vi "SYST_PRES.vi"(0 "VISA IN":refnum<visa-resource-name>, 5 "error in":errorcluster) -> (14 "VISA Out":refnum<visa-resource-name>, 19 "error out":errorcluster)   [LabVIEW 2018, in "PNA-X.lvlib"] (continued)
 Count (PWIN ONLY) \n1758\n\n<value> (String) Parameter Value for the specified stage 3 parameter. Use the query form \nto return the minimum and maximum values for the specified parameter. \nExamples SENS:IF:FILT:STAGe3:PAR \"C\",64 \nsense2:if:filter:stage3:parameter \"d\",0.5E-6 \nQuery Syntax SENSe<cnum>:IF:FILTer:STAGE3:PARameter? <p> \nreturns the current parameter value \nSENSe<cnum>:IF:FILTer:STAGE3:PARameter? <p>,Min \nreturns the minimum parameter value. \nSENSe<cnum>:IF:FILTer:STAGE3:PARameter? <p>,Max \nreturns the maximum parameter value. \nExamples SENS:IF:FILT:STAGe3:PAR? \"C\" \nsense2:if:filter:stage3:parameter? \"d\",min \nReturn Type Numeric \nDefault RECT: C = 1 \nPWIN: C=1E6, P=10ms, D=50us, W=50us, R=7 \nTUKEY: C=1 \nSENSe<cnum>:IF:FILTer:STAGE3:PCATalog? \n(Read-only) Returns a list of the available parameters for the currently selected filter type. \nCritical Note \nParameters \n<cnum> Existing channel number. If unspecified, <cnum> is set to 1. \nExamples SENS:IF:FILT:STAGe3:PCAT? \nsense2:if:filter:stage3:pcatalog? \nReturn Type String \nDefault Not Applicable \nSENSe<cnum>:IF:FREQuency:AUTO <bool> \n1759\n\n(Read-Write) Sets and returns the method for specifying the way the IF Frequency is determined. \nCritical Note \nParameters \n<cnum> Existing channel number. If unspecified, <cnum> is set to 1. \n<bool> (Boolean) \nON (or 1) - Automatic. PNA determines the setting for the IF frequency. \nOFF (or 0) - Manual. Use SENS:IF:FREQ to set the frequency. \nExamples SENS:IF:FREQ:AUTO 1 \nsense2:if:frequency:auto 0 \nQuery Syntax SENSe<cnum>:IF:FREQuency:AUTO? \nReturn Type Boolean \nDefault ON \nSENSe<cnum>:IF:FREQuency[:VALue] <value> \n(Read-Write) Sets and returns the IF frequency for ALL receiver paths being used for the specified \nchannel. To set this frequency, SENS:IF:FREQ:AUTO must be set to OFF (Manual). \nAlso returns the maximum and minimum allowable frequency settings. \nCritical Note \nParameters \n<cnum> Existing channel number. If unspecified, <cnum> is set to 1. \n<value> (Numeric) Frequency value. \nExamples SENS:IF:FREQ \nsense2:if:frequency \nQuery Syntax SENSe<cnum>:IF:FREQuency? \n'returns the current frequency setting \nSENSe<cnum>:IF:FREQuency? Max \n'returns the maximum allowable frequency setting \nSENSe<cnum>:IF:FREQuency? Min \n'returns the minimum allowable frequency setting \nReturn Type Numeric \nDefault 9 MHz \n1760\n\nLast Modified: \n18-Jan-2007 MX New topic \n1761\n\nSense:Mixer Commands \nPerforms Mixer setup and configuration. \nClick on a blue keyword to view the command details. \nSee Also \nExample Programs \nLearn about the Frequency Converter Application \nSynchronizing the PNA and Controller \nSCPI Command Tree \nSENSe<ch>:MIXer:APPLy \n(Write only) Applies the mixer setup settings and turns the channel ON. (Performs the same function \nas the Apply button on the mixer setup dialog box). \nParameters \n<ch> Any existing channel number. If unspecified, value is set to 1 \nExamples SENS:MIX:APPL \nQuery Syntax Not Applicable \nDefault Not Applicable \n1762\n\nSENSe<ch>:MIXer:AVOidspurs <bool> \n(Read Write) Sets and returns the state of the avoid spurs feature. Learn more about avoid spurs. \nParameters \n<ch> Any existing channel number. If unspecified, value is set to 1 \n<bool> Avoid spurs state. Choose from \n0 - Avoid spurs OFF \n1 - Avoid spurs ON \nExamples SENS:MIX:AVO \nsense2:mixer:avoidspurs 1 \nQuery Syntax SENSe<ch>:MIXer:AVOidspurs? \nReturn Type Boolean \nDefault 0 (OFF) \nSENSe<ch>:MIXer:CALCulate <char> \n(Write only) Calculates the Input, IF, or Output frequencies of the mixer setup and updates the \nchannel settings. \nParameters \n<ch> Any existing channel number. If unspecified, value is set to 1 \n<char> Mixer port to be calculated. Choose from: \n1763\n\n<char> 1st or only stage \nrequires: \nIn addition, 2nd stage \nrequires: \nINPUT \nOutput Start and Stop \nfrequencies \nLO frequency \nOutput sideband (High or \nLow) \nIF Start and Stop \nfrequencies \n2nd LO frequency \nIF sideband (High or Low) \nBoth NA \nIF Start and Stop \nfrequencies \nBoth LO frequencies \nOUTPUT \nInput Start and Stop \nfrequencies \nLO frequency \nOutput sideband (High or \nLow) \nIF Start and Stop \nfrequencies \n2nd LO frequency \nIF sideband (High or Low) \nLO_1 \nInput Start and Stop \nfrequencies \nOutput frequency \nOutput sideband (High or \nLow) \nIF Start and Stop \nfrequencies \n2nd LO frequency \nIF sideband (High or Low) \nLO_2 NA Input Start and stop \nfrequencies \n1st LO start and stop \nfrequencies \nOutput frequency \nIF sideband(High or Low \nOutput sideband(High or \nLow) \nExamples SENS:MIX:CALC Output \nQuery Syntax Not Applicable \nDefault Not Applicable \nSENSe<ch>:MIXer:LOAD <name> \n1764\n\n(Write-only) Loads a previously-configured mixer attributes file (.mxr) \nParameters \n<ch> Any existing channel number. If unspecified, value is set to 1. \n<name> Path and file name (including .mxr extension) to load. \nExamples SENSe:MIXer:LOAD \"C:\\Program Files\\Agilent\\Network \nAnalyzer\\Documents\\Mixer\\MyMixer.mxr\" \nDefault Not Applicable \nSENSe<ch>:MIXer:SAVE <name> \n(Write-only) Saves the settings for the mixer/converter test setup to a mixer attributes file. \nParameters \n<ch> Any existing channel number. If unspecified, value is set to 1. \n<name> Path and file name (including .mxr extension) to save. \nExamples SENSe:MIXer:SAVE \"C:\\Program Files\\Agilent\\Network \nAnalyzer\\Documents\\Mixer\\MyMixer.mxr\" \nDefault Not Applicable \nSENSe<ch>:MIXer:STAGe <n> \n(Read-Write) Number of IF stages of the mixer. \nParameters \n<ch> Any existing channel number. If unspecified, value is set to 1. \n<n> Number of stages. Choose either 1 or 2 \nExamples SENSe:MIX:STAG 2 \nSENSe:MIXer:STAGE 1 \nQuery Syntax SENSe<ch>:MIXer:STAGe? \nReturn Type Numeric \nDefault 1 \nSENSe<ch>:MIXer:IF:FREQuency:DENominator <num> \n1765\n\n(Read-Write) Sets or returns the denominator value of the IF Fractional Multiplier. \nParameters \n<ch> Any existing channel number. If unspecified, value is set to 1. \n<num> Denominator value. \nExamples SENSe:MIX:IF:FREQ:DEN 5 \nSENSe2:MIXer:IF:FREQ:DENominator 4 \nQuery Syntax SENSe<ch>:MIXer:IF:FREQuency:DENominator? \nReturn Type Numeric \nDefault Not Applicable \nSENSe<ch>:MIXer:IF:FREQuency:FIXed <num> \n(Read-Write) Sets or returns the fixed frequency of the IF.. \nParameters \n<ch> Any existing channel number. If unspecified, value is set to 1. \n<num> Frequency. \nExamples SENSe:MIXer:IF:FREQ:FIXed 1e9 \nSENSe2:MIXer:IF:FREQ:FIXed 1000000000 \nQuery Syntax SENSe<ch>:MIXer:IF:FREQuency:FIXed? \nReturn Type Numeric \nDefault Not Applicable \nSENSe<ch>:MIXer:IF:FREQuency:NUMerator <num> \n(Read-Write) Sets or returns the numerator value of the IF Fractional Multiplier. \nParameters \n<ch> Any existing channel number. If unspecified, value is set to 1. \n<num> Numerator value of the IF fractional multiplier \nExamples SENSe:MIX:IF:FREQ:NUM 4 \nSENSe2:MIXer:IF2:FREQ:NUMerator 3 \nQuery Syntax SENSe<ch>:MIXer:IF:FREQuency:NUMerator? \nReturn Type Numeric \nDefault Not Applicable \n1766\n\nSENSe<ch>:MIXer:IF:FREQuency:SIDeband <char> \n(Read-Write) Sets or returns the value of the IF sideband. \nParameters \n<ch> Any existing channel number. If unspecified, value is set to 1. \n<char> Sideband value. Choose from \nLOW - Low or Difference (-) \nHIGH - High or Sum (+) \nExamples SENS:MIX:IF:FREQ:SIDE LOW \nSENSe2:MIXer:IF:FREQ:SIDEband HIGH \nQuery Syntax SENSe<ch>:MIXer:IF:FREQuency:SIDeband? \nReturn Type Character \nDefault LOW \nSENSe<ch>:MIXer:IF:FREQuency:STARt <num> \n(Read-Write) Sets or returns the IF start frequency value of the mixer. \nParameters \n<ch> Any existing channel number. If unspecified, value is set to 1. \n<num> IF Start Frequency value \nExamples SENS:MIX:IF:FREQ:STAR 1e9 \nSENSe2:MIXer:IF:FREQ:STARt 1000000000 \nQuery Syntax SENSe<ch>:MIXer:IF:FREQuency:STARt? \nReturn Type Numeric \nDefault Not Applicable \nSENSe<ch>:MIXer:IF:FREQuency:STOP <num>\n1767\n\n(Read-Write) Sets or returns the stop frequency value of the mixer IF frequency. \nParameters \n<ch> Any existing channel number. If unspecified, value is set to 1. \n<num> IF Stop Frequency value \nExamples SENS:MIX:IF:FREQ:STOP 2e9 \nSENSe2:MIXer:IF:FREQ:STOP 2000000000 \nQuery Syntax SENSe<ch>:MIXer:IF:FREQuency:STOP? \nReturn Type Numeric \nDefault Not Applicable \nSENSe<ch>:MIXer:INPut:FREQuency:DENominator <value> \n(Read-Write) Sets or returns the denominator value of the Input Fractional Multiplier. \nParameters \n<ch> Any existing channel number. If unspecified, value is set to 1. \n<value> Input denominator value. \nExamples SENS:MIX:INP:FREQ:DEN 5 \nSENS2:MIXer:INPut:FREQ:DENominator 4 \nQuery Syntax SENSe<ch>:MIXer:INPut:FREQuency:DENominator? \nReturn Type Numeric \nDefault Not Applicable \nSENSe<ch>:MIXer:INPut:FREQuency:FIXed<value> \n(Read-Write) Sets or returns the fixed frequency of the input. \nParameters \n<ch> Any existing channel number. If unspecified, value is set to 1. \n<value> Input frequency. \nExamples SENSe:MIXer:INPut:FREQ:FIXed 1e9 \nSENSe2:MIXer:INPut:FREQ:FIXed 1000000000 \nQuery Syntax SENSe<ch>:MIXer:INPut:FREQuency:FIXed? \nReturn Type Numeric \nDefault Not Applicable \n1768\n\nSENSe<ch>:MIXer:INPut:FREQuency:MODE <char> \n(Read-Write) Sets or returns the Input sweep mode. \nParameters \n<ch> Any existing channel number. If unspecified, value is set to 1. \n<char> Input sweep mode. Choose either FIXED or SWEPT \nExamples SENS:MIX:INP:FREQ:MODE FIXED \nSENSe2:MIXer:INP:FREQ:MODE swept \nQuery Syntax SENSe<ch>:MIXer:INPut:FREQuency:MODE? \nReturn Type Character \nDefault Fixed \nSENSe<ch>:MIXer:INPut:FREQuency:NUMerator <value> \n(Read-Write) Sets or returns the numerator value of the Input Fractional Multiplier. \nParameters \n<ch> Any existing channel number. If unspecified, value is set to 1. \n<value> Input numerator value. \nExamples SENS:MIX:INP:FREQ:NUM 3 \nSENSe2:MIXer:INPut:FREQ:NUMerator 1 \nQuery Syntax SENSe<ch>:MIXer:INPut:FREQ:NUMerator? \nReturn Type Numeric \nDefault Not Applicable \nSENSe<ch>:MIXer:INPut:FREQuency:STARt <value> \n1769\n\n(Read-Write) Sets or returns the Input start frequency value of the mixer. \nParameters \n<ch> Any existing channel number. If unspecified, value is set to 1. \n<value> Input Start frequency \nExamples SENS:MIX:INP:FREQ:STAR 1e9 \nSENSe2:MIXer:INPut:FREQ:STARt 1000000000 \nQuery Syntax SENSe<ch>:MIXer:INPut:FREQuency:STARt? \nReturn Type Numeric \nDefault Not Applicable \nSENSe<ch>:MIXer:INPut:FREQuency:STOP <value> \n(Read-Write) Sets or returns the Input stop frequency value of the mixer. \nParameters \n<ch> Any existing channel number. If unspecified, value is set to 1. \n<value> Input stop frequency \nExamples SENS:MIX:INP:FREQ:STOP 2e9 \nSENSe2:MIXer:INPut:FREQ:STOP 2000000000 \nQuery Syntax SENSe<ch>:MIXer:INPut:FREQuency:STOP? \nReturn Type Numeric \nDefault Not Applicable \nSENSe<ch>:MIXer:INPut:POWer <value> \n(Read-Write) Sets or returns the value of the Input Power. \nParameters \n<ch> Any existing channel number. If unspecified, value is set to 1. \n<value> Input power in dBm. \nExamples SENS:MIX:INP:POW 9 \nSENSe2:MIXer:INPut:POWer 5 \nQuery Syntax SENSe<ch>:MIXer:INPut:POWer? \nReturn Type Numeric \nDefault Not Applicable \n1770\n\nSENSe<ch>:MIXer:INPut:POWer:USENominal <bool> \n(Read-Write) Toggles the Nominal Incident Power setting ON and OFF. This setting is ONLY to be \nused with SMC measurements, not VMC. Learn more about Nominal Incident Power. \nParameters \n<ch> Any existing channel number. If unspecified, value is set to 1. \n<value> (boolean) - Nominal Incident Power State. Choose from: \nTrue (1) - Turn nominal incident power ON \nFalse (0) - Turn nominal incident power OFF \nExamples SENS:MIX:INP:POW:USEN 1 \nSENSe2:MIXer:INPut:POWer:USENominal false \nQuery Syntax SENSe<ch>:MIXer:INPut:POWer:USENominal? \nReturn Type Boolean \nDefault False \nSENSe<ch>:MIXer:LO<n>:FREQuency:DENominator <value> \n(Read-Write) Sets or returns the denominator value of the LO Fractional Multiplier. \nParameters \n<ch> Any existing channel number. If unspecified, value is set to 1. \n<n> LO stage number. Choose 1 or 2. \n<value> LO denominator. \nExamples SENS:MIX:LO:FREQ:DEN 5 \nSENSe2:MIXer:LO2:FREQ:DENominator 4 \nQuery Syntax SENSe<ch>:MIXer:LO<n>:FREQuency:DENominator? \nReturn Type Numeric \nDefault 1 \nSENSe<ch>:MIXer:LO<n>:FREQuency:FIXed <value> \n1771\n\n(Read-Write) Sets or returns the fixed frequency of the specified mixer LO. \nParameters \n<ch> Any existing channel number. If unspecified, value is set to 1. \n<n> LO stage number. Choose 1 or 2 \n<value> LO frequency. \nExamples SENS:MIX:LO:FREQ:FIX 1e9 \nSENSe2:MIXer:LO2:FREQ:FIXed 1000000000 \nQuery Syntax SENSe<ch>:MIXer:LO<n>:FREQuency:FIXed? \nReturn Type Numeric \nDefault Not Applicable \nSENSe<ch>:MIXer:LO<n>:FREQuency:ILTI <bool> \n(Read-Write) Specifies whether to use the Input frequency that is greater than the LO or less than \nthe LO. To learn more, see the mixer setup dialog box help. \nParameters \n<ch> Any existing channel number. If unspecified, value is set to 1. \n<n> LO stage number. Choose 1 or 2 \n<bool> True (1) - Use the Input that is Greater than the specified LO. \nFalse (0) - Use the Input that is Less than the specified LO. \nExamples SENS:MIX:LO1:FREQ:ILTI 1 \nsense2:mixer:lo2:frequency:ilti true \nQuery Syntax SENSe<ch>:MIXer:LO<n>:FREQuency:ILTI? \nReturn Type Boolean \nDefault False \nSENSe<ch>:MIXer:LO<n>:FREQuency:MODE <char> \n1772\n\n(Read-Write) Sets or returns the LO sweep mode. \nParameters \n<ch> Any existing channel number. If unspecified, value is set to 1. \n<n> LO stage number. Choose 1 or 2 \n<char> LO sweep mode. Choose either FIXED or SWEPT \nExamples SENS:MIX:LO:FREQ:MODE FIXED \nSENSe2:MIXer:LO2:FREQ:MODE swept \nQuery Syntax SENSe<ch>:MIXer:LO<n>:FREQuency:MODE? \nReturn Type Character \nDefault Fixed \nSENSe<ch>:MIXer:LO<n>:FREQuency:NUMerator <value> \n(Read-Write) Sets or returns the numerator value of the LO Fractional Multiplier. \nParameters \n<ch> Any existing channel number. If unspecified, value is set to 1. \n<n> LO stage number. Choose 1 or 2 \n<value> LO Numerator. \nExamples SENS:MIX:LO:FREQ:NUM 5 \nSENSe2:MIXer:LO2:FREQ:NUMerator 4 \nQuery Syntax SENSe<ch>:MIXer:LO<n>:FREQuency:NUMerator? \nReturn Type Numeric \nDefault Not Applicable \nSENSe<ch>:MIXer:LO<n>:FREQuency:STARt <value> \n1773\n\n(Read-Write) Sets or returns the LO start frequency value. \nParameters \n<ch> Any existing channel number. If unspecified, value is set to 1. \n<n> LO stage number. Choose 1 or 2 \n<value> LO Start Frequency in Hertz. \nExamples SENS:MIX:LO:FREQ:STAR 5E9 \nQuery Syntax SENSe<ch>:MIXer:LO<n>:FREQuency:STARt? \nReturn Type Numeric \nDefault Not Applicable \nSENSe<ch>:MIXer:LO<n>:FREQuency:STOP <value> \n(Read-Write) Sets or returns the LO stop frequency value. \nParameters \n<ch> Any existing channel number. If unspecified, value is set to 1. \n<n> LO stage number. Choose 1 or 2 \n<value> LO Stop Frequency in Hertz. \nExamples SENS:MIX:LO:FREQ:STOP 5E9 \nQuery Syntax SENSe<ch>:MIXer:LO<n>:FREQuency:STOP? \nReturn Type Numeric \nDefault Not Applicable \nSENSe<ch>:MIXer:LO<n>:NAME <value> \n1774\n\n(Read-Write) Sets or returns the name of the previously-configured external LO source. The external \nLO source must be configured and calibrated manually; there are no programming commands to \naccomplish this. The source must also be properly connected. \nParameters \n<ch> Any existing channel number. If unspecified, value is set to 1. \n<n> LO stage number. Choose 1 or 2. \n<value> External LO source name \nExamples SENS:MIX:LO:NAME \"MySource\" \nQuery Syntax SENSe<ch>:MIXer:LO<n>:NAME? \nReturn Type String \nDefault Not Controlled \nSENSe<ch>:MIXer:LO<n>:POWer <value> \n(Read-Write) Sets or returns the value of the LO Power. \nParameters \n<ch> Any existing channel number. If unspecified, value is set to 1. \n<n> LO stage. Choose 1 or 2 \n<value> LO Power in dBm \nExamples SENS:MIX:LO:POW 9 \nQuery Syntax SENSe<ch>:MIXer:LO<n>:POWer? \nReturn Type Numeric \nDefault Not Applicable \nSENSe<ch>:MIXer:OUTPut:FREQuency:FIXed <value> \n1775\n\n(Read-Write) Sets or returns the output fixed frequency of the mixer. \nParameters \n<ch> Any existing channel number. If unspecified, value is set to 1. \n<value> Output fixed frequency in Hertz. \nExamples SENS:MIX:OUTP:FREQ:FIX 5e9 \nQuery Syntax SENSe<ch>:MIXer:OUTPut:FREQuency:FIXed? \nReturn Type Numeric \nDefault Not Applicable \nSENSe<ch>:MIXer:OUTPut:FREQuency:MODE <char> \n(Read-Write) Sets or returns the Output sweep mode. \nParameters \n<ch> Any existing channel number. If unspecified, value is set to 1. \n<char> Output sweep mode. Choose either FIXED or SWEPT \nExamples SENS:MIX:OUT:FREQ:MODE FIXED \nSENSe2:MIXer:OUTput:FREQuency:MODE swept \nQuery Syntax SENSe<ch>:MIXer:OUTPut:FREQuency:MODE? \nReturn Type Character \nDefault Fixed \nSENSe<ch>:MIXer:OUTPut:FREQuency:SIDeband <value> \n1776\n\n(Read-Write) Sets or returns the value of the output sideband. \nParameters \n<ch> Any existing channel number. If unspecified, value is set to 1. \n<value> Boolean Sideband value. Choose from \nLOW - Low or Difference (-) \nHIGH - High or Sum (+) \nExamples SENS:MIX:OUTP:FREQ:SIDe LOW \nSENSe2:MIXer:OUTPut:FREQ:SIDeband HIGH \nQuery Syntax SENSe<ch>:MIXer:OUTPut:FREQuency:SIDeband? \nReturn Type Character \nDefault LOW \nSENSe<ch>:MIXer:OUTPut:FREQuency:STARt <value> \n(Read-Write) Sets or returns the Output start frequency of the mixer. \nParameters \n<ch> Any existing channel number. If unspecified, value is set to 1. \n<value> Output start frequency \nExamples SENS:MIX:OUTP:FREQ:STAR 1e9 \nSENSe2:MIXer:OUTPut:FREQ:STARt 1000000000 \nQuery Syntax SENSe<ch>:MIXer:OUTPut:FREQuency:STARt? \nReturn Type Numeric \nDefault Not Applicable \nSENSe<ch>:MIXer:OUTPut:FREQuency:STOP <value> \n1777\n\n(Read-Write) Sets or returns the Output stop frequency of the mixer. \nParameters \n<ch> Any existing channel number. If unspecified, value is set to 1. \n<value> Output stop frequency \nExamples SENS:MIX:OUTP:FREQ:STOP 1e9 \nSENSe2:MIXer:OUTPut:FREQ:STOP 1000000000 \nQuery Syntax SENSe<ch>:MIXer:OUTPut:FREQuency:STOP? \nReturn Type Numeric \nDefault Not Applicable \n1778\n\nSense:Multiplexer Commands \nControls External Test Sets (N44xx, E5091A, and Special Opts). \nClick on a blue keyword to view the command details. \nRed commands are superseded. \nSee Also \nSee an example program using these commands. \nLearn about External Test Set Control \nSynchronizing the PNA and Controller \nSCPI Command Tree \nSENSe:MULTiplexer<id>:ADDRess <address> \n(Read-Write) Sets and returns the address for the external test set at the specified ID. This command \nshould be immediately preceded by the SENSe:MULT:TYPE command. \nParameters \n<id> Id of the external test set. If unspecified, Id is assumed to be 1. Must be \npreviously set by the SENSe:MULT:TYPE command. \n<address> Integer The test set address. \nFor a GPIB test set (N44xx and some specials), this is the GPIB address. \nFor a test set I/O test set (some specials), it is the position of the test set in the chain \n(starting at 0). \nFor USB test sets (E5091A), the address is set by DIP switches on the rear panel. \n1779\n\nExamples SENS:MULT1:TYPE \"Z5623A_K66\" ' use K66 test set, and reference it \nthrough ID 1 \nSENS:MULT1:ADDR 0 ' first test set in sequence \n' All subsequent commands using SENS:MULT1 will refer to this \ntest set \nQuery Syntax SENSe:MULTiplexer<id>:ADDRess? \nReturn Type Numeric \nDefault Not Applicable \nSENSe<cnum>:MULTiplexer<id>:ALLPorts <string> \n(Read-Write) Sets or gets the port selections for all available ports on the specified channel. \nParameters \n<cnum> Any existing channel number. If unspecified, value is set to 1. \n<id> Id of the external test set. If unspecified, Id is assumed to be 1. Must be \npreviously set by the SENSe:MULT:TYPE command. \n<string> Comma-separated list of port selections, one for each port. Each port selection \nmust correspond to one of the values returned by SENS:MULT:PORT:CAT?. \nDo NOT include + and - . \nExamples ' for channel 5 and test set 1, set port 1 to T1, \n' port 2 to A, port 3 to R2+, port 4 to R3-. \nSENS5:MULT1:ALLP \"T1,A,R2,R3 \" \nQuery Syntax SENSe<cnum>:MULTiplexer<id>:ALLPorts? \nReturn Type STRING \nDefault Not Applicable \nSENSe:MULTiplexer:CATalog? \n(Read-Only) Returns a comma-separated list of the external test sets models that are currently \nsupported. Choose one of these items to send SENS:MULT1:TYPE. \nExamples SENS:MULT:CAT? \nReturn Type String \nDefault Not Applicable \n1780\n\nSENSe:MULTiplexer<id>:COUNt? \n(Read-Only) Returns the total number of ports of the specified test set. \nReturns 0 if no test set is connected (GPIB test sets only). \nParameters \n<id> Id of the external test set. If unspecified, Id is assumed to be 1. Must be \npreviously set by the SENSe:MULT:TYPE command. \nExamples SENS:MULT1:COUN? \nsense:multiplexer2:count? \nReturn Type Numeric \nDefault Not Applicable \nSENSe:MULTiplexer<id>:DISPlay[:STATe] <bool> \n(Read-Write) Turns ON and OFF the display of the test set control status bar. This status bar indicates \nthe test set that is being controlled and the current port mappings. This setting is turned ON \nautomatically when the test set is enabled. \nParameters \n<id> Id of the external test set. If unspecified, Id is assumed to be 1. Must be \npreviously set by the SENSe:MULT:TYPE command. \n<bool> ON(1) Turns ON the display. \nOFF (0) Turns OFF the display. \nExamples SENS:MULT1:DISP 1 \nsense:multiplexer2:display:state on \nQuery Syntax SENSe:MULTiplexer<id>:DISPlay[:STATe]? \nReturn Type Boolean \nDefault OFF (0) \nSENSe:MULTiplexer<id>:INCount? \n1781\n\n(Read-Only) Returns the number of input ports for the specified test set. \nFor test sets such as the E5091A that do NOT use jumper cables to route the stimulus and response signals, \nthis command returns the number of test set ports that can be connected to the PNA. \nFor test sets that DO use jumper cables to route the stimulus and response signals, such as the N44xx, the \nreturn value is not valid. \nParameters \n<id> Id of the external test set. If unspecified, Id is assumed to be 1. Must be \npreviously set by the SENSe:MULT:TYPE command. \nExamples SENS3:MULT1:INC? ' returns the number of input ports for test \nset 1 on channel 3 \nReturn Type Numeric \nDefault Not Applicable \nSENSe<cnum>:MULTiplexer:LABel <string> \n(Read-Write) Sets and returns the display label for the testset on the specified channel. The label \nappears in a status bar at the bottom of the PNA display when SENS:MULT:DISP is set to TRUE. \nParameters \n<cnum> Any existing channel number. If unspecified, value is set to 1. \n<string> Display label text. \nExamples SENS3:MULT:LAB 'High-power output' \nQuery Syntax SENSe<cnum>:MULTiplexer:LABel? \nReturn Type String \nDefault Not Applicable \nSENSe<cnum>:MULTiplexer<id>:OUTPut[:DATa] <num> \n1782\n\n(Read-Write) Sets or returns the control line value for the specified channel. \nParameters \n<cnum> Any existing channel number. If unspecified, value is set to 1. \n<id> Id of the external test set. If unspecified, Id is assumed to be 1. Must be \npreviously set by the SENSe:MULT:TYPE command. \n<numr> An integer specifying the decimal value of the control line. Values are obtained \nby adding weights from the following table that correspond to individual lines. \nHIGH =1; LOW=0. \nLine Weight \n1 1 \n2 2 \n3 4 \n4 8 \n5 16 \n6 32 \n7 64 \n8 128 \n0 - Sets all lines low \n255 - Sets all lines high \nExamples SENS3:MULT1:OUTP 48 'For test set 1 on channel 3, sets lines 5 \nand 6 to HIGH state; all other lines are set to LOW state. \nQuery Syntax SENSe<cnum>:MULTiplexer<id>:OUTPut[:DATa]? \nReturn Type Numeric \nDefault Not Applicable \nSENSe:MULTiplexer<id>:PORT<pnum>CATalog? \n1783\n\n(Read-Only) Returns a comma-separated list of valid port selections for the specified port. \nParameters \n<id> Id of the external test set. If unspecified, Id is assumed to be 1. Must be \npreviously set by the SENSe:MULT:TYPE command. \n<pnum> Integer - Input port number for which to return valid Output port selections. \nRead the number of input ports for the test set using SENS:MULT:INCount? \nExamples SENS:MULT1:PORT3:CAT? ' returns the valid port selections for \nport 3 \nReturn Type String \nDefault Not Applicable \nSENSe<cnum>:MULTiplexer<id>:PORT<logi>SELect <phys> \n(Write-Only) Sets and returns a port mapping for a single port. If this command creates a conflict with \nan existing port, the PNA will resolve the conflict. \nNote: This command is currently not supported for the Z5623AK44. \nParameters \n<cnum> Channel number of the measurement. If unspecified, value is set to 1. \n<id> Id of the external test set. If unspecified, Id is assumed to be 1. Must be \npreviously set by the SENSe:MULT:TYPE command. \n<logi> Integer - Logical port number. \n<string> String - Physical port number. \nExamples SENS:MULT1:PORT3:SEL \"4\" 'sets logical port 3 to physical port \n4. \nReturn Type String \nDefault Not Applicable \nSENSe:MULTiplexer<id>:STATe <bool> \n1784\n\n(Read-Write) Enables and disables (ON/OFF) the port mapping and control line output of the \nspecified test set. \nIf the specified test set is not connected or not ON, then setting State ON will report an error. All other \nproperties can be set when the test set is not connected. \nWhen this command is set to ON, then the display of the test set status bar (SENS:MULT:DISP) is \nalso set to ON. \nParameters \n<id> Id of the external test set. If unspecified, Id is assumed to be 1. Must be \npreviously set by the SENSe:MULT:TYPE command. \n<bool> ON(1) Enables test set control. \nOFF (0) Disables test set control. \nExamples SENS:MULT1:STAT 1 \nsense2:multiplexer2:state on \nQuery Syntax SENSe<cnum>:MULTiplexer<id>:STATe? \nReturn Type Boolean \nDefault OFF (0) \nSENSe<cnum>:MULTiplexer<id>:TSET9:OUTPut[:DATA] <data> Superseded \nNote: This command is replaced with SENS:MULT:OUTP \n(Read-Write) Sets the control lines of the specified E5091A. Control lines, provided through a \nE5091A front panel connector, are used to control external equipment such as a part handler. See your \nE5091A documentation to learn more about control lines. \nParameters \n<cnum> Channel number of the measurement. If unspecified, value is set to 1. \n<id> Id of the E5091A test set. Choose from 1 or 2. Learn how to set ID value. \n<data> Data value used to set control lines. Values are obtained by adding weights \nfrom the following table that correspond to individual lines. HIGH =1; \nLOW=0. \n1785\n\nLine Weight \n1 1 \n2 2 \n3 4 \n4 8 \n5 16 \n6 32 \n7 64 \n8 128 \n0 - Sets all lines low \n255 - Sets all lines high \nExamples 'The following sets line 3 and 4 high. All other lines low. \nSENS:MULT1:TSET9:OUTP 12 \nQuery Syntax SENSe<cnum>:MULTiplexer<id>:TSET9:OUTPut[:DATA]? \nReturn Type Numeric \nDefault 0 \nSENSe<cnum>:MULTiplexer<id>:TSET9:PORT1 <char> Superseded \nNote: This command is replaced with SENS:MULT:ALLPorts which sets ALL ports to the specified \noutputs. \n(Read-Write) Switches Port 1 of the specified E5091A to one of the available outputs. \nParameters \n<cnum> Any existing channel number; if unspecified, value is set to 1. \n<id> Id of the E5091A test set. Choose from 1 or 2. Learn how to set ID value. \n<char> Output port to be switched to. Choose from: \nA\nT1 - (If Port 2 already is connected to T1, then Port 2 will be switched to T2.) \nExamples SENS:MULT1:TSET9:PORT1 A \nQuery Syntax SENSe<cnum>:MULTiplexer<id>:TSET9:PORT1? \n1786\n\nReturn Type Character \nDefault A \nSENSe<cnum>:MULTiplexer<id>:TSET9:PORT2 <char> Superseded \nNote: This command is replaced with SENS:MULT:ALLPorts which sets ALL ports to the specified \noutputs. \n(Read-Write) Switches Port 2 of the specified E5091A to one of the available outputs. \nParameters \n<cnum> Any existing channel number; if unspecified, value is set to 1. \n<id> Id of the E5091A test set. Choose from 1 or 2. Learn how to set ID value. \n<char> Output port to be switched to. Choose from: \nT1 - If Port 1 already is connected to T1, then Port 1 will be switched to A. \nT2 \nExamples SENS:MULT1:TSET9:PORT2 T2 \nQuery Syntax SENSe<cnum>:MULTiplexer<id>:TSET9:PORT2? \nReturn Type Character \nDefault T1 \nSENSe<cnum>:MULTiplexer<id>:TSET9:PORT3 <char> Superseded \nNote: This command is replaced with SENS:MULT:ALLPorts which sets ALL ports to the specified \noutputs. \n(Read-Write) Switches Port 3 of the specified E5091A to one of the available outputs. \nParameters \n<cnum> Any existing channel number; if unspecified, value is set to 1. \n<id> Id of the E5091A test set. Choose from 1 or 2. Learn how to set ID value. \n<char> Output port to be switched to. Choose from: \nR1 (R1+) \nR2 (R2+) \n1787\n\nR3 (R3+) If option 007 (7port), R2 is selected. \nExamples SENS:MULT1:TSET9:PORT3 R2 \nQuery Syntax SENSe<cnum>:MULTiplexer<id>:TSET9:PORT3? \nReturn Type Character \nDefault R1 \nSENSe<cnum>:MULTiplexer<id>:TSET9:PORT4 <char> Superseded \nNote: This command is replaced with SENS:MULT:ALLPorts which sets ALL ports to the specified \noutputs. \n(Read-Write) Switches Port 4 of the specified E5091A to one of the available outputs. \nParameters \n<cnum> Any existing channel number; if unspecified, value is set to 1. \n<id> Id of the E5091A test set. Choose from 1 or 2. Learn how to set ID value. \n<char> Output port to be switched to. Choose from: \nR1 (R1-) \nR2 (R2-) \nR3 (R3-) If option 007 (7port), R2 is selected. \nExamples SENS:MULT1:TSET9:PORT4 R2 \nQuery Syntax SENSe<cnum>:MULTiplexer<id>:TSET9:PORT4? \nReturn Type Character \nDefault R1 \nSENSe:MULTiplexer<id>:TYPe <name> \n1788\n\n(Read-Write) Loads a configuration file for the specified type of external test set. \nThis command should be immediately followed by the SENSe:MULT:ADDRess command. \nParameters \n<name> \nString The name of the type of test set. Must be one of the items in the list \nreturned by the SENSe:MULT:CATalog? query. \n<id> Id of the external test set. Set by this command. Use consecutive values starting \nat 1. \nExamples SENS:MULT1:TYPE \"Z5623AK66\" ' use K66 test set, and reference \nit through ID 1 \nQuery Syntax SENSe:MULTiplexer<id>:TYPe? \nReturn Type String \nDefault Not Applicable \n1789\n\nSense:Offset Commands \nSets the offset frequency functions, causing the stimulus and response frequencies to be different. \nClick on a blue keyword to view the command details. \nSee Also \nExample Programs \nLearn about Frequency Offset \nSynchronizing the PNA and Controller \nSCPI Command Tree \nSENSe<cnum>:OFFSet:CW <bool> \n(Read-Write) Turns stimulus CW Override mode ON or OFF. Use this setting to establish a fixed \n(CW) stimulus frequency while measuring the Response over a swept frequency range. \nParameters \n<cnum> Any existing channel number. If unspecified, value is set to 1 \n<bool> ON (or 1) - turns CW override ON. \nOFF (or 0) - turns CW overide OFF. \nExamples SENS:OFFS:CW ON \nsense2:offset:cw off \nQuery Syntax SENSe<cnum>:OFFSet:CW? \nReturn Type Boolean \nDefault OFF \nSENSe<cnum>:OFFSet:DIVisor <num> \n1790\n\n(Read-Write) Specifies (along with the multiplier) the value to multiply by the stimulus. \nParameters \n<cnum> Any existing channel number. If unspecified, value is set to 1 \n<num> Divisor value. Range is 1 to 1000 \nExamples SENS:OFFS:DIV 3 \nsense2:offset:divisor 2 \nQuery Syntax SENSe<cnum>:OFFSet:DIVisor? \nReturn Type Numeric \nDefault 1 \nSENSe<cnum>:OFFSet:MULTiplier <num> \n(Read-Write) Specifies (along with the divisor) the value to multiply by the stimulus. \nParameters \n<cnum> Any existing channel number. If unspecified, value is set to 1 \n<num> Multiplier value. Range is +/- 1000. Negative multipliers cause the stimulus to \nsweep in decreasing direction. For mixer measurements, this would be for \nsetups requiring the RF frequency to be less than LO frequency \nExamples SENS:OFFS:MULT 2 \nsense2:offset:multiplier 4 \nQuery Syntax SENSe<cnum>:OFFSet:MULTplier? \nReturn Type Numeric \nDefault 1 \nSENSe<cnum>:OFFSet:OFFSet <num> \n1791\n\n(Read-Write) Specifies an absolute offset frequency in Hz. For mixer measurements, this would be \nthe LO frequency. \nParameters \n<cnum> Any existing channel number. If unspecified, value is set to 1 \n<num> Offset frequency. Range is +/- 1000 GHz. Offsets can be positive or negative \nExamples SENS:OFFS:OFFS 1GHz \nsense2:offset:offset 1e9 \nQuery Syntax SENSe<cnum>:OFFSet:OFFSet? \nReturn Type Numeric \nDefault 0 Hz \nSENSe<cnum>:OFFSet:STARt? \n(Read-Only) Returns the response start frequency \nParameters \n<cnum> Any existing channel number. If unspecified, value is set to 1 \nExamples SENS:OFFS:STAR? \nsense2:offset:start? \nReturn Type Numeric \nDefault Not applicable \nSENSe<cnum>:OFFSet:[STATe] <bool> \n(Read-Write) Enables Frequency Offset Mode on ALL measurements that are present on the active \nchannel. This immediately causes the source and receiver to tune to separate frequencies. The receiver \nfrequencies are specified with the other SENS:OFFSet commands. To make the stimulus settings use \nthe SENS:FREQ commands. \nTip: To avoid unnecessary errors, first make other offset frequency settings, then set Frequency Offset \nON. \nParameters \n<cnum> Any existing channel number. If unspecified, value is set to 1 \n<bool> ON (or 1) - turns Frequency Offset ON. \nOFF (or 0) - turns Frequency Offset OFF. \n1792\n\nExamples SENS:OFFS ON \nsense2:offset:state off \nQuery Syntax SENSe<cnum>:OFFSet:[STATe]? \nReturn Type Boolean \nDefault OFF (0) \nSENSe<cnum>:OFFSet:STOP? \n(Read-Only) Returns the response stop frequency. \nParameters \n<cnum> Any existing channel number. If unspecified, value is set to 1 \nExamples SENS:OFFS:STOP \nsense2:offset:stop \nReturn Type Numeric \nDefault Not applicable \n1793\n\nSense:Path:Configuration Commands \nControls the path configuration settings. \nClick on a blue keyword to view the command details. \nSee Also \nExample Programs \nLearn about Path Configuration \nSynchronizing the PNA and Controller \nSCPI Command Tree \nSENSe:PATH:CONFiguration:CATalog? \n(Read-only) Returns a list of configuration names stored in the PNA. \nExamples SENS:PATH:CONF:CAT? \nReturn Type Comma-separated list of double-quoted strings \nDefault Not Applicable \nSENSe:PATH:CONFiguration:DELete <string> \n1794\n\n(Write-only) Deletes the specified configuration name from the PNA. The factory configurations cannot be \ndeleted. This is the only method of distinguishing a factory configuration from a user-named configuration. \nParameters \n<string> Configuration name to be deleted. \nExamples SENS:PATH:CONF:DEL \"MyMixer\" \nReturn Type Not Applicable \nDefault Not Applicable \nSENSe:PATH:CONFiguration:DTEXt <string> \n(Read-Write) Write and read descriptive text associated with the configuration. This text is displayed in the path \nconfiguration dialog. Text is generally used to describe external connections that must be made manually to \ncomplete the configuration setup. \nParameters \n<string> Descriptive text enclosed in quotes. Double quotes are not allowed within the descriptive \ntext. \nExamples SENS:PATH:CONF:DTEX \"Connect J1 jumper on the rear panel.\" \nQuery Syntax SENSe<ch>:PATH:CONFiguration:DTEXt? \nReturn Type String \nDefault Not Applicable \nSENSe<ch>:PATH:CONFiguration:ELEMent:CATalog? \n1795\n\n(Read-only) Returns the names of configurable elements as a comma-delimited list of strings. \nSee a list of configurable elements and settings for various PNA models. \nParameters \n<ch> Any existing channel number; if unspecified, value is set to 1. \nExamples SENS:PATH:CONF:ELEM:CAT? \n'returns \n�Combiner�, �Src1�, �Src2� \nDefault Not Applicable \nSENSe<ch>:PATH:CONFiguration:ELEMent[:STATe] <elem>, <setting> \n(Read-Write) Write or read the setting of a specified element in the current configuration. \nSee a list of configurable elements and settings for various PNA models. \nParameters \n<ch> Any existing channel number; if unspecified, value is set to 1. \n<elem> Name of the element for which a setting is to be made. \n<setting> Element setting. Use SENS:PATH:CONF:ELEM:VAL:CAT? to return a list of valid \nsettings for the specified element. \nExamples SENS:PATH:CONF:ELEM \"Combiner\",\"Normal\" \nQuery Syntax SENSe<ch>:PATH:CONFiguration:ELEMent? \"Combiner\" \nReturns the current state of the Combiner element. \nReturn Type String \nDefault Not applicable \nSENSe<ch>:PATH:CONFiguration:ELEMent:VALue:CATalog? <element> \n1796\n\n(Read-only) Returns the list of valid settings that can be used with the specified element. \nSee a list of configurable elements and settings for various PNA models. \nParameters \n<ch> Any existing channel number; if unspecified, value is set to 1. \n<element> String. Element name for which to return valid settings. \nExamples SENS:PATH:CONF:ELEM:VAL:CAT? \"Combiner\" \n'returns \"Normal\", \"Reversed\" \nDefault Not Applicable \nSENSe<ch>:PATH:CONFiguration:NAME? \n(Read-only) Returns the name of the current configuration only if NO individual element settings had been \nchanged since selecting or storing a configuration. When element settings change, the path configuration name is \ncleared. \nParameters \n<ch> Any existing channel number; if unspecified, value is set to 1. \nExamples SENS:PATH:CONF:NAME? \n'returns \"Default\" \nReturn Type String \nDefault Not Applicable \nSENSe<ch>:PATH:CONFiguration:SELect <string> \n1797\n\n(Write only) Loads the named configuration onto the specified channel. \nUse SENS:PATH:CONF:CAT? to return the configuration names that are stored on the PNA. \nParameters \n<ch> Any existing channel number; if unspecified, value is set to 1. \n<string> Configuration name. \"Default\" is the default factory configuration. \nExamples SENS:PATH:CONF:SEL 'default' \nsense2:path:configuration:select \"MyMixer\" \nQuery Syntax Not Applicable \nDefault \"Default\" \nSENSe<ch>:PATH:CONFiguration:STORe <name> \n(Write only) Saves the path configuration currently associated with channel <ch> to the specified configuration \nname. \nParameters \n<ch> Any existing channel number; if unspecified, value is set to 1. \n<name> String. Configuration name. Factory configurations can NOT be overwritten. Specifying \nthe name of a pre-defined factory configuration will result in an error. \nExamples SENS:PATH:CONF:STOR \"MyMixer\" \nQuery Syntax Not Applicable \nDefault Not Applicable \nLast Modified: \n14-Dec-6 MX New Topic \n1798\n\nSense:Power Command \nLearn about Receiver Attenuation \nSENSe<cnum>:POWer:ATTenuation <recvr>,<num> \n(Read-Write) Sets the attenuation level for the specified receiver. \nNote: Attenuation cannot be set with Sweep Type set to Power \nParameters \n<cnum> Any existing channel number. If unspecified, value is set to 1 \n<recvr> Receiver to get attenuation. Choose from: \nARECeiver - receiver A \nBRECeiver - receiver B \nReceiver attenuation can not be set using logical receiver notation. \n<num> Choose from: \n0 to 35 dB - in 5 dB steps \nIf a number other than these is entered, the analyzer will select the next lower \nvalid value. For example, if 19.9 is entered for <num> the analyzer will switch \nin 15 dB attenuation. \nExamples SENS:POW:ATT AREC,10 \nsense2:power:attentuation breceiver,30 \nQuery Syntax SENSe<cnum>:POWer:ATTenuation? <rec> \nReturn Type Numeric \nDefault 0 \n1799\n\nSense:Pulse Commands \nConfigures the 5 pulse generators in the PNA-X. \nClick on a blue keyword to view the command details. \nPulse Definitions \nD = Delay; the time before each pulse begins \nW = Width; the time the pulse is ON \nP = Period; one complete pulse cycle \nDuty Cycle = W/P \nImportant: If D + W is greater than P, then undefined PNA behavior results. There is NO error \nmessage or warning. \nSee Also \nPNA-X IF Path Block diagram \nSENS:IF configuration commands \nExample Programs \nPNA-X Pulse Application \nSynchronizing the PNA and Controller \nSCPI Command Tree \n1800\n\nSENSe<ch>:PULSe<n>:DELay <value> \n(Read-Write) Sets the pulse delay. The amount of time before a new pulse begins. \nSee Pulse Definition diagram. \nParameters \n<ch> Any existing channel number; if unspecified, value is set to 1. \n<n> Pulse generator number. Choose from 0 to 4. \n0 is the generator that pulses the ADC. \n<value> Delay value in seconds. Choose a value from about 33ns to about 70 seconds. \nExamples SENS:PULS:DEL .5 \nQuery Syntax SENSe<ch>:PULSe<n>:DELay? \nReturn Type Numeric \nDefault 0 \nSENSe<ch>:PULSe<n>:DINCrement <value> \n(Read-Write) Sets the pulse delay increment. The delay increments with each pulse by the <value> \namount. \nFor example, in this diagram the delay starts as 1. On the second pulse, delay=2. On the third pulse, \ndelay=3. \nImportant: If D + W is greater than P, then undefined PNA behavior results. There is NO error \nmessage or warning. Delay includes the incremented value. \nThis is useful for pulse profiling. \nSee Pulse Definition diagram. \nParameters \n<ch> Any existing channel number; if unspecified, value is set to 1. \n1801\n\n<n> Pulse generator number. Choose from 0 to 4. \n0 is the generator that pulses the ADC. \n<value> Delay increment value in seconds. \nExamples SENS:PULS:DINC .5 \nQuery Syntax SENSe<ch>:PULSe<n>:DINCrement? \nReturn Type Numeric \nDefault 0 \nSENSe<ch>:PULSe:PERiod <value> \n(Read-Write) Sets the pulse-period (1/PRF) for ALL pulse generators. \nThe resolution of the period is 16.667nS. \nSee Pulse Definition diagram. \nParameters \n<ch> Any existing channel number; if unspecified, value is set to 1. \n<value> Pulse period in seconds. Choose a value from about 33ns to about 70 seconds. \nExamples SENS:PULS:PERiod .5 \nQuery Syntax SENSe<ch>:PULSe:PERiod? \nReturn Type Numeric \nDefault 1e-3 sec \nSENSe<ch>:PULSe<n>:STATe <bool> \n1802\n\n(Read-Write) Turns the pulse output ON and OFF. \nParameters \n<ch> Any existing channel number; if unspecified, value is set to 1. \n<n> Pulse generator number. Choose from 0 to 4. \n0 is the generator that pulses the ADC. \n<bool> ON (or 1) - turns pulse output ON. \nOFF (or 0) - turns pulse output OFF. \nExamples SENS:PULS:STAT 1 \nQuery Syntax SENSe<ch>:PULSe:STATe? \nReturn Type Boolean \nDefault OFF \nSENSe<ch>:PULSe<n>:WIDTh <value> \n(Read-Write) Sets the pulse width. The amount of time that the pulse is ON. \nSee Pulse Definition diagram. \nParameters \n<ch> Any existing channel number; if unspecified, value is set to 1. \n<n> Pulse generator number. Choose from 0 to 4. \n0 is the generator that pulses the ADC. \n<value> Pulse width in seconds. Choose a value from about 33ns to about 70 seconds. \nExamples SENS:PULS:WIDT .5 \nQuery Syntax SENSe<ch>:PULSe<n>:WIDTh? \nReturn Type Numeric \nDefault 1e-4 sec \nLast Modified: \n2-Jan-2007 MX New topic \n1803\n\nSense:Roscillator Command \nLearn about the Reference Osc. \nSENSe:ROSCillator:SOURce? \n(Read-only) Applying a signal to the Reference Oscillator connector automatically sets the Reference \nOscillator to EXTernal. This command allows you to check that it worked. \nEXT is returned when a signal is present at the Reference Oscillator connector. \nINT is returned when NO signal is present at the Reference Oscillator connector. \nExamples SENS:ROSC:SOUR? \nsense:roscillator:source? \nReturn Type Character \nDefault Not applicable \n1804\n\nSense:Segment Commands \nDefines the segment sweep settings. Enable segment sweep with SENS:SWE:TYPE SEGMent. \nClick on a blue keyword to view the command details. \nSee Also \nExample Programs \nLearn about Segment Sweep \nSynchronizing the PNA and Controller \nSCPI Command Tree \nSENSe<cnum>:SEGMent<snum>:ADD \n(Write-only) Adds a segment. \nParameters \n<cnum> Any existing channel number. If unspecified, value is set to 1 \n<snum> Segment number to add. If unspecified, value is set to 1. Segment numbers must \nbe sequential. If a new number is added where one currently exists, the existing \nsegment and those following are incremented by one. \nExamples Two Segments exist (1 and 2). The following command will add a new segment (1). The \nexisting (1 and 2) will become (2 and 3) respectively. \nSENS:SEGM1:ADD \nsense2:segment1:add \nQuery Syntax Not applicable. Use Sense:Segment:Count to determine the number of segments in a \ntrace. \nDefault Not Applicable \nSENSe<cnum>:SEGMent:ARBitrary <ON | OFF> \n1805\n\n(Read-Write) Enables you to setup a segment sweep with arbitrary frequencies. The start and stop \nfrequencies of each segment can overlap other segments. Also, each segment can have a start \nfrequency that is greater than its stop frequency which causes a reverse sweep over that segment. \nLearn more about Arbitrary Segment Sweep. \nParameters \n<cnum> Any existing channel number. If unspecified, value is set to 1. \n<ON | OFF> ON (or 1) - Allows the setup of arbitrary segment sweep. \nOFF (or 0) - Prevents the setup of arbitrary segment sweep. \nExamples SENS:SEGM:ARB ON \nsense2:segment:arbitrary off \nQuery Syntax SENSe<cnum>:SEGMent:ARBitrary? \nReturn Type Boolean (1 = ON, 0 = OFF) \nDefault OFF \nSENSe<cnum>:SEGMent<snum>:BWIDth[:RESolution] <num> \n(Read-Write) Sets the IF Bandwidth for the specified segment. First set \nSENS:SEGM:BWIDth:CONTrol ON. All subsequent segments that are added assume the \nnew IF Bandwidth value. \nParameters \n<cnum> Any existing channel number. If unspecified, value is set to 1 \n<snum> Segment number to modify. Choose any existing segment number. \n<num> IF Bandwidth in Hz. The list of valid IF Bandwidths is different depending on \nthe PNA model. (Click to see the lists.) If an invalid number is specified, the \nanalyzer will round up to the closest valid number. \nNote: This command will accept MIN or MAX instead of a numeric parameter. \nSee SCPI Syntax for more information. \nExamples SENS:SEGM:BWID 1KHZ \nsense2:segment2:bwidth:resolution max \nQuery Syntax SENSe<cnum>:SEGMent<snum>:BWIDth[:RESolution]? \nReturn Type Numeric \nDefault See Preset IFBW for your PNA model. \nSENSe<cnum>:SEGMent:BWIDth[:RESolution]:CONTrol <ON | OFF> \n1806\n\n(Read-Write) Specifies whether the IF Bandwidth resolution can be set independently for each \nsegment. \nParameters \n<cnum> Any existing channel number. If unspecified, value is set to 1 \n<ON | OFF> ON (or 1) - turns Bandwidth control ON. Bandwidth can be set for each \nsegment \nOFF (or 0) - turns Bandwidth control OFF. Use channel bandwidth setting \nExamples SENS:SEGM:BWID:CONT ON \nsense2:segment:bwidth:control off \nQuery Syntax SENSe<cnum>:SEGMent:BWIDth[:RESolution]:CONTrol? \nReturn Type Boolean (1 = ON, 0 = OFF) \nDefault OFF \nSENSe<cnum>:SEGMent:COUNt? \n(Read-only) Queries the number of segments that exist in the specified channel. \nParameters \n<cnum> Any existing channel number. If unspecified, value is set to 1 \nExamples SENS:SEGM:COUNt? \nsense2:segment:count? \nReturn Type Numeric \nDefault 1 segment \nSENSe<cnum>:SEGMent<snum>:DELete \n(Write-only) Deletes the specified sweep segment. When ALL segments are deleted, Sweep Mode \n(SENS:SWE:MODE) is automatically set to Linear because there are no segments to sweep. \n<cnum> Any existing channel number. If unspecified, value is set to 1 \n<snum> Number of the segment to delete. If unspecified, value is set to 1 \nExamples SENS:SEGM:DEL \nsense2:segment2:delete \nQuery Syntax Not applicable \nDefault Not Applicable \n1807\n\nSENSe<cnum>:SEGMent:DELete:ALL \n(Write-only) Deletes all sweep segments. When this command is executed, Sweep Mode \n(SENS:SWE:MODE) is automatically set to Linear because there are no segments to sweep. \nParameters \n<cnum> Any existing channel number. If unspecified, value is set to 1 \nExamples SENS:SEGM:DEL:ALL \nsense2:segment:delete:all \nQuery Syntax Not applicable \nDefault Not Applicable \nSENSe<cnum>:SEGMent<snum>:FREQuency:CENTer <num> \n(Read-Write) Sets the Center Frequency for the specified segment. The Frequency Span of the \nsegment remains the same. The Start and Stop Frequencies change accordingly. \nNote: All previous segment's Start and Stop Frequencies that are larger than the new Start Frequency \nare changed to the new Start Frequency. All following segment's start and stop frequencies that are \nsmaller than the new Stop Frequency are changed to the new Stop Frequency. \nParameters \n<cnum> Any existing channel number. If unspecified, value is set to 1 \n<snum> Segment number to modify. Choose any existing segment number. \n<num> Center Frequency in Hz. Choose any number between the minimum and \nmaximum frequency of the analyzer. \nNote: This command will accept MIN or MAX instead of a numeric parameter. \nSee SCPI Syntax for more information. \nExamples SENS:SEGM:FREQ:CENT 1MHZ \nsense2:segment2:frequency:center 1e9 \nQuery Syntax SENSe<cnum>:SEGMent<snum>:FREQuency:CENTer? \nReturn Type Numeric \nDefault Stop Frequency of the previous segment. If first segment, start frequency of the \nanalyzer. \nSENSe<cnum>:SEGMent<snum>:FREQuency:SPAN <num> \n1808\n\n(Read-Write) Sets the Frequency Span for the specified segment. The center frequency of the segment \nremains the same. The start and stop frequencies change accordingly. \nNote: All previous segment's Start and Stop Frequencies that are larger than the new Start Frequency \nare changed to the new Start Frequency. All following segment's start and stop frequencies that are \nsmaller than the new Stop Frequency are changed to the new Stop Frequency. \nParameters \n<cnum> Any existing channel number. If unspecified, value is set to 1 \n<snum> Segment number to modify. Choose any existing segment number. \n<num> Frequency Span in Hz. Choose any number between the minimum and \nmaximum frequency of the analyzer. \nNote: This command will accept MIN or MAX instead of a numeric parameter. \nSee SCPI Syntax for more information. \nExamples SENS:SEGM:FREQ:SPAN 1MHZ \nsense2:segment2:frequency:span max \nQuery Syntax SENSe<cnum>:SEGMent<snum>:FREQuency:SPAN? \nReturn Type Numeric \nDefault If first segment, frequency span of the analyzer. Otherwise 0. \nSENSe<cnum>:SEGMent<snum>:FREQuency:START <num> \n(Read-Write) Sets the Start Frequency for the specified sweep segment. \nNotes \nAll other segment Start and Stop Frequency values that are larger than this frequency are changed to \nthis frequency. \nTo return the start and stop frequency of the entire sweep (all segments), Use SENS:FREQ:STARt? \nand SENS:FREQ:STOP? \nParameters \n<cnum> Any existing channel number. If unspecified, value is set to 1 \n<snum> Segment number to modify. Choose any existing segment number. \n<num> Start Frequency in Hz. Choose any number between the minimum and \nmaximum frequency of the analyzer. \nNote: This command will accept MIN or MAX instead of a numeric parameter. \n1809\n\nSee SCPI Syntax for more information. \nExamples SENS:SEGM:FREQ:STAR 1MHZ \nsense2:segment2:frequency:start minimum \nQuery Syntax SENSe<cnum>:SEGMent<snum>:FREQuency:STARt? \nReturn Type Numeric \nDefault Stop Frequency of the previous segment. If first segment, start frequency of the \nanalyzer. \nSENSe<cnum>:SEGMent<snum>:FREQuency:STOP <num> \n(Read-Write) Sets the Stop Frequency for the specified sweep segment. \nNotes \nAll other segment Start and Stop Frequency values that are larger than this frequency are changed to \nthis frequency. \nTo return the start and stop frequency of the entire sweep (all segments), Use SENS:FREQ:STARt? \nand SENS:FREQ:STOP? \nParameters \n<cnum> Any existing channel number. If unspecified, value is set to 1 \n<snum> Segment number to modify. Choose any existing segment number. \n<num> Stop Frequency in Hz. Choose any number between the minimum and \nmaximum frequency of the analyzer. \nNote: This command will accept MIN or MAX instead of a numeric parameter. \nSee SCPI Syntax for more information. \nExamples SENS:SEGM:FREQ:STOP 1MHZ \nsense2:segment2:frequency:stop maximum \nQuery Syntax SENSe<cnum>:SEGMent<snum>:FREQuency:STOP? \nReturn Type Numeric \nDefault If first segment, stop frequency of the analyzer. Otherwise, start frequency of the \nsegment. \nSENSe<cnum>:SEGMent<snum>:POWer[<port>][:LEVel] <num> \n1810\n\n(Read-Write) Sets the Port Power level for the specified sweep segment. First set \nSENS:SEGM:POW:CONTrol ON. \nWhen port power is Coupled, setting port power for one port will apply port power for all source \nports. \nAll subsequent segments that are added assume the new Power Level value. \nParameters \n<cnum> Any existing channel number. If unspecified, value is set to 1 \n<snum> Segment number to modify. Choose any existing segment number. \n<port> Port number of the source. If unspecified, value is set to 1. \n<num> Power level. \nNote: The range of settable power values depends on the PNA model and if \nsource attenuators are installed. To determine the range of values, send \nSOUR:POW? MAX and SOUR:POW? MIN. (SOUR:POW:ATT:AUTO must \nbe set to ON). \nActual achievable leveled power depends on frequency. \nExamples SENS:SEGM:POW 0 \nsense2:segment2:power1:level -10 \nQuery Syntax SENSe<cnum>:SEGMent<snum>:POWer[<port>][:LEVel]? \nReturn Type Numeric \nDefault 0 \nSENSe<cnum>:SEGMent:POWer[:LEVel]:CONTrol <ON | OFF> \n1811\n\n(Read-Write) Specifies whether Power Level can be set independently for each segment. \nParameters \n<cnum> Any existing channel number. If unspecified, value is set to 1 \n<ON | OFF> ON (or 1) - turns Power Level control ON. Power level can be set for each \nsegment. \nOFF (or 0) - turns Power Level control OFF. Use the channel power level \nsetting. \nExamples SENS:SEGM:POW:CONT ON \nsense2:segment:power:level:control off \nQuery Syntax SENSe<cnum>:SEGMent:POWer[:LEVel]:CONTrol? \nReturn Type Boolean (1 = ON, 0 = OFF) \nDefault OFF \nSENSe<cnum>:SEGMent<snum>[:STATe] <ON | OFF> \n(Read-Write) Turns the specified sweep segment ON or OFF. At least ONE segment must be ON or \nSweep Mode is automatically set to Linear. \nParameters \n<cnum> Any existing channel number. If unspecified, value is set to 1 \n<snum> Segment number to be turned ON or OFF \n<ON | OFF> ON (or 1) - turns segment ON. \nOFF (or 0) - turns segment OFF. \nExamples SENS:SEGM ON \nsense2:segment2:state off \nQuery Syntax SENSe<cnum>:SEGMent<snum>[:STATe]? \nReturn Type Boolean (1 = ON, 0 = OFF) \nDefault OFF \nSENSe<cnum>:SEGMent<snum>:SWEep:POINts <num> \n1812\n\n(Read-Write) Sets the number of data points for the specified sweep segment. \nParameters \n<cnum> Any existing channel number. If unspecified, value is set to 1 \n<snum> Any existing segment number. If unspecified, value is set to 1 \n<num> Number of points in the segment. The total number of points in all segments \ncannot exceed 16001. A segment can have as few as 1 point. \nNote: This command will accept MIN or MAX instead of a numeric parameter. \nSee SCPI Syntax for more information. \nExamples SENS:SEGM:SWE:POIN 51 \nsense2:segment2:sweep:points maximum \nQuery Syntax SENSe<cnum>:SEGMent<snum>:SWEep:POINts? \nReturn Type Numeric \nDefault 21 \nSENSe<cnum>:SEGMent<snum>:SWEep:TIME <num> \n(Read-Write) Sets the time the analyzer takes to sweep the specified sweep segment. \nParameters \n<cnum> Any existing channel number. If unspecified, value is set to 1 \n<snum> Any existing segment number. \n<num> Sweep time in seconds. Choose a number between 0 and 100 \nNote: This command will accept MIN or MAX instead of a numeric \nparameter. See SCPI Syntax for more information. \nExamples SENS:SEGM:SWE:TIME 1ms \nsense2:segment2:sweep:time .001 \nQuery Syntax SENSe<cnum>:SEGMent<snum>:SWEep:TIME? \nReturn Type Numeric \nDefault Not Applicable \nSENSe<cnum>:SEGMent:SWEep:TIME:CONTrol <ON | OFF> \n1813\n\n(Read-Write) Specifies whether Sweep Time can be set independently for each sweep segment. \nParameters \n<cnum> Any existing channel number. If unspecified, value is set to 1 \n<ON | OFF> ON (or 1) - turns Sweep Time control ON. Sweep Time can be set for each \nsegment. \nOFF (or 0) - turns Sweep Time control OFF. Uses the channel Sweep Time \nsetting. \nExamples SENS:SEGM:SWE:TIM:CONT ON \nsense2:segment:sweep:time:control off \nQuery Syntax SENSe<cnum>:SEGMent:SWEep:TIME:CONTrol? \nReturn Type Boolean (1 = ON, 0 = OFF) \nDefault OFF \nSENSe<cnum>:SEGMent<snum>:X:SPACing <char> \n(Read-Write) Sets X-axis spacing ON or OFF \nParameters \n<cnum> Any existing channel number. If unspecified, value is set to 1 \n<snum> Any existing segment number. (This parameter is ignored) \n<char> LINear - turns X-axis point spacing OFF \nOBASe - turns X-axis point spacing ON \nExamples SENS:SEGM:X:SPACing LIN \nsense2:segment1:spacing obase \nQuery Syntax SENSe<cnum>:SEGMent<snum>:X:SPACing? \nReturn Type Character \nDefault LINear \n1814\n\nSense:Sweep Commands \nSpecifies the sweep functions of the analyzer. \nClick on a blue keyword to view the command details. \nSee Also \nExample Programs \nExample Triggering the PNA using SCPI \nLearn about Sweeping \nSynchronizing the PNA and Controller \nSCPI Command Tree \nNote: All of the commands in this block will accept MIN or MAX instead of a numeric parameter. \nAlso, kHZ, MHz, and GHz are accepted as suffixes/units. \nSee SCPI Syntax for more information. \nSENSe<cnum>:SWEep:DWELl <num> \n(Read-Write) Sets the dwell time between each sweep point. \nDwell time is ONLY available with SENSe:SWEep:GENeration set to STEPped; It is Not available in \nANALOG. \nSending dwell = 0 is the same as setting SENS:SWE:DWEL:AUTO ON. Sending a dwell time > 0 sets \nSENS:SWE:DWEL:AUTO OFF. \nParameters \n<cnum> Any existing channel number. If unspecified, value is set to 1 \n<num> Dwell time in seconds. \nSee Note \nExamples SENS:SWE:DWEL .1 \nsense2:sweep:dwell min \n1815\n\nQuery Syntax SENSe<cnum>:SWEep:DWELl? \nReturn Type Numeric \nDefault 0 - (Note: dwell time set to 0 is the same as dwell:auto ON) \nSENSe<cnum>:SWEep:DWELl:AUTO <ON | OFF> \n(Read-Write) Specifies whether or not to automatically calculate and set the minimum possible dwell time. Setting \nAuto ON has the same effect as setting dwell time to 0. \nParameters \n<cnum> Any existing channel number. If unspecified, value is set to 1 \n<ON | OFF> ON (or 1) - turns dwell ON. \nOFF (or 0) - turns dwell OFF. \nExamples SENS:SWE:DWEL:AUTO ON \nsense2:sweep:dwell:auto off \nQuery Syntax SENSe<cnum>:SWEep:DWELl:AUTO? \nReturn Type Boolean (1 = ON, 0 = OFF) \nDefault ON \nSENSe<cnum>:SWEep:GENeration <char> \n(Read-Write) Sets sweep as Stepped or Analog. \nParameters \n<cnum> Any existing channel number. If unspecified, value is set to 1 \n<char> Choose from: \nSTEPped - source frequency is CONSTANT during measurement of eah displayed \npoint. More accurate than ANALog. Dwell time can be set in this mode. \nANALog - source frequency is continuously RAMPING during measurement of each \ndisplayed point. Faster than STEPped. Sweep time (not dwell time) can be set in this \nmode. \nExamples SENS:SWE:GEN STEP \nsense2:sweep:generation analog \nQuery Syntax SENSe<cnum>:SWEep:GENeration? \nReturn Type Character \nSENSe<cnum>:SWEep:GROups:COUNt <num>\n1816\n\nDefault Analog \nSENSe<cnum>:SWEep:GROups:COUNt <num> \n(Read-Write) Sets the trigger count (groups) for the specified channel. Set trigger mode to group after setting this \ncount. \nParameters \n<cnum> Any existing channel number. If unspecified, value is set to 1 \n<num> Count (groups) number. Choose any number between: \n1 and 2e6 (1 is the same as single trigger) \nExamples SENS:SWE:GRO:COUN 10 \nsense2:sweep:groups:count 50 \nQuery Syntax SENSe<cnum>:SWEep:GROups:COUNt? \nReturn Type Numeric \nDefault 1 \nSENSe<cnum>:SWEep:MODE <char> \n(Read-Write) Sets the number of trigger signals the specified channel will ACCEPT. \nSee Triggering the PNA Using 
